vi "Untitled 3.vi"() -> ()   [LabVIEW 2018]
panel:
  out "s? t:f":string
  in  "Slide":dbl(slide) scale=0.0..100.0
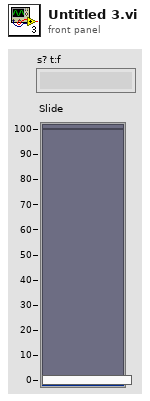
[diagram p1: front panel]
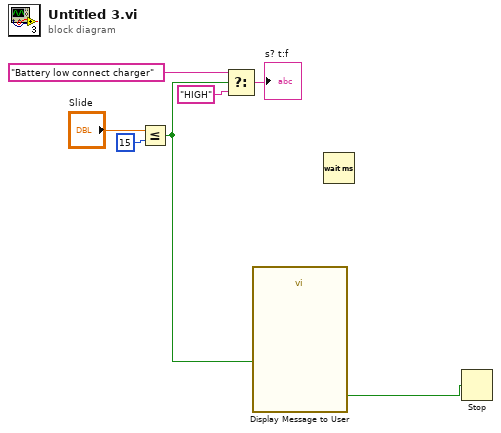
[diagram p0: block diagram]
diagram:
  n1 = Less Or Equal?(x="Slide", y=15) -> (x <= y?=w1:bool)
  n2 = Select(t="Battery low connect charger", s=w1, f="HIGH") -> (s? t:f=→"s? t:f":string)
  n3 = call "Display Message to User"("Enable"=w1) -> ("OK"=w2:bool)  [unwired: 9 in, 1 out]
  n4 = Wait (ms)() -> ()  [unwired: 1 in, 1 out]
  n5 = Stop(stop? (T)=w2) -> ()
